vi "Actor Core.vi"(8 "error in":errorcluster, 11 "Meter in":refnum<class "Meter.lvclass">) -> (0 "error out":errorcluster, 3 "Actor out":refnum<class "Actor.lvclass">)   [LabVIEW 2018, in "Meter Actor.lvlib" / "Meter.lvclass"]
doc: "(<B>Filename</B>: Actor Framework.lvlib:Actor.lvclass:Actor Core.vi)\n\nReceives messages to the actor, reacts to them, and initiates any error handling that may shut the actor down.\n\nDescendant classes may override this VI to append parallel tasks for the actor to complete while it handles messages. Overrides use the Call Parent Method node."
uses:
  Meter.lvclass
  C:/Users/Administrator/Desktop/2018LabVIEW EMS/EMS Generic Actor/EMS Generic/EMS Generic.lvclass
  <vilib>/ActorFramework/Actor/Actor.lvclass
  EMS Generic Actor/EMS Generic/EMS Generic.lvclass/EMS Generic.ctl
  <vilib>/ORNL/CSEISMIC DDS/CSEISMIC DDS Base/CSEISMIC DDS.lvclass/CSEISMIC DDS.ctl
  <vilib>/ORNL/CSEISMIC DDS/CSEISMIC DDS Base/Accessors/Write DDS Reference.vi
  <vilib>/ORNL/CSEISMIC DDS/CSEISMIC DDS Base/Accessors/Read DDS Reference.vi
  <vilib>/ORNL/CSEISMIC DDS/DDS Reader/DDS Reader.lvclass
  C:/Program Files (x86)/National Instruments/LabVIEW 2018/vi.lib/ORNL/CSEISMIC DDS/CSEISMIC DDS Base/CSEISMIC DDS.lvclass
  <vilib>/ORNL/CSEISMIC DDS/CSEISMIC DDS Base/Error Handler.vi
  Device DDS Communications Framework/Device DDS Communications/Device DDS Communications.lvclass
  EMS Generic Actor/EMS Generic/EMS Generic.lvclass
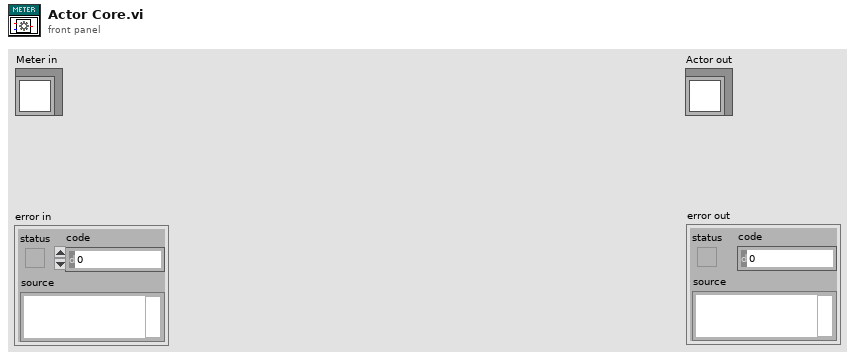
[diagram p1: front panel]
types:
  T1 = typedef "CSEISMIC DDS.lvlib/CSEISMIC DDS.lvclass/DeviceID.ctl" = string
  T2 = typedef "CSEISMIC DDS.lvlib/CSEISMIC DDS.lvclass/Meter_Measurement.ctl" = cluster{"DeviceID":T1, "Voltage":dbl[], "Current":dbl[], "RealPower":dbl[], "ReactivePower":dbl[], "LineConfig":u8[], "Frequency":dbl}
  T3 = typedef "LVDDS_library.lvlib/DDS Sample Info.ctl" = cluster{"DDS_SampleStateKind":enum32{"DDS_INVALID_SAMPLE_STATE", "DDS_READ_SAMPLE_STATE", "DDS_NOT_READ_SAMPLE_STATE"}, "DDS_ViewStateKind":enum32{"DDS_INVALID_SAMPLE_STATE", "DDS_NEW_VIEW_STATE", "DDS_NOT_NEW_VIEW_STATE"}, "DDS_InstanceStateKind":enum32{"DDS_INVALID_STATE", "DDS_ALIVE_INSTANCE_STATE", "DDS_NOT_ALIVE_DISPOSED_INSTANCE_STATE", "", "DDS_NOT_ALIVE_NO_WRITERS_INSTANCE_STATE"}, "sec":i32, "nanosec":u32, "valid_data":bool}
  T4 = typedef "CSEISMIC DDS.lvlib/CSEISMIC DDS.lvclass/Meter_Info.ctl" = cluster{"DeviceID":T1, "LineConfig":u8[], "NominalVoltage(V)":dbl}
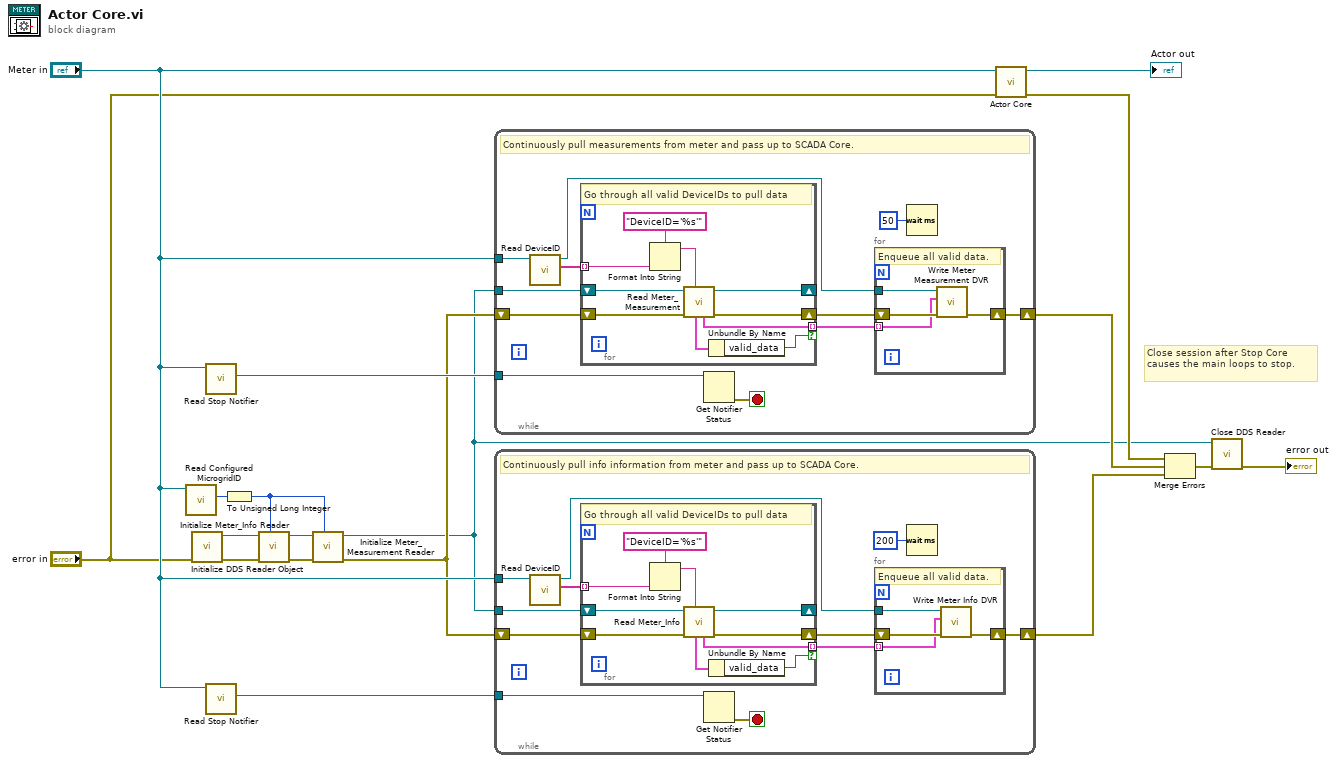
[diagram p0: block diagram]
diagram:
  # "Close session after Stop Core causes the main loops to stop."
  n1 = call "Read Configured MicrogridID.vi"("EMS Generic in"="Meter in") -> ("Microgrid ID"=w18:u8)  [unwired: 8 in, 2 out]
  n2 = call <vilib>:"Initialize DDS Reader Object.vi"("error in"="error in") -> ("error out"=w12:errorcluster, "DDS Reader out"=w11:refnum<class "DDS Reader.lvclass">)  [unwired: 9 in]
  n3 = call "Read Stop Notifier.vi"("EMS Generic in"="Meter in") -> ("stop"=w14:refnum<notifier>)  [unwired: 9 in, 1 out]
  n4 = call "Read Stop Notifier.vi"("EMS Generic in"="Meter in") -> ("stop"=w7:refnum<notifier>)  [unwired: 9 in, 1 out]
  n5 = To Unsigned Long Integer(number=w18) -> (unsigned 32bit integer=w9:u32)
  n6 = call <vilib>:"Initialize Meter_Info Reader.vi"("MicrogridID"=w9, "error in"=w12, "DDS Reader in"=w11) -> ("error out"=w13:errorcluster, "DDS Reader out"=w10:refnum<class "DDS Reader.lvclass">)  [unwired: 7 in]
  n7 = call <vilib>:"Initialize Meter_Measurement Reader.vi"("MicrogridID"=w9, "error in"=w13, "DDS Reader in"=w10) -> ("error out"=w5:errorcluster, "DDS Reader out"=w4:refnum<class "DDS Reader.lvclass">)  [unwired: 7 in]
  n8 = while {
    tunnel: w14 -> [w29]
    shift-right: [w28] -> w17
    shift-left: w5 -> [w23]
    tunnel: "Meter in" -> [w25]
    tunnel: w4 -> [w22]
    stop <- w27 stop-if-true
    # "Continuously pull measurements from meter and pass up to SCADA Core."
    n9 = call-dynamic "Read DeviceID.vi"("Device DDS Communications in"=w25) -> ("DeviceID"=w24:T1[], "Device DDS Communications out"=w19:refnum<class "Meter.lvclass">)  [unwired: 9 in]
    n10 = for {
      shift-right: [w42] -> _
      shift-left: w22 -> [w43]
      shift-right: [w41] -> w21
      shift-left: w23 -> [w40]
      tunnel: w24 -> [w38] mode=indexing
      tunnel: [w35] -> w20 mode=indexing if=w34
      # "Go through all valid DeviceIDs to pull data"
      n11 = Format Into String(format string="DeviceID='%s'", w38) -> (resulting string=w37:string)  [unwired: 2 in, 1 out]
      n12 = call <vilib>:"Read Meter_Measurement.vi"("Query condition"=w37, "error in"=w40, "DDS Reader in"=w43) -> ("error out"=w41:errorcluster, "DDS Reader out"=w42:refnum<class "DDS Reader.lvclass">, "data"=w35:T2, "DDS Sample Info"=w36:T3)  [unwired: 5 in]
      n13 = Unbundle By Name(w36) -> ("valid_data"=w34:bool)
    }
    n14 = Get Notifier Status(notifier=w29) -> (error out=w27:errorcluster)  [unwired: 1 in, 4 out]
    n15 = for {
      shift-right: [w32] -> w28
      shift-left: w21 -> [w33]
      tunnel: w20 -> [w31] mode=indexing
      tunnel: w19 -> [w30]
      # "Enqueue all valid data."
      n16 = call "Write Meter Measurement DVR.vi"("error in"=w33, "Meter_Measurement"=w31, "EMS Generic in"=w30) -> ("error out"=w32:errorcluster)  [unwired: 7 in, 1 out]
    }
    n17 = Wait (ms)(milliseconds to wait=u32 50) -> ()  [unwired: 1 out]
  }
  n18 = while {
    tunnel: w7 -> [w54]
    shift-right: [w53] -> w3
    shift-left: w5 -> [w48]
    tunnel: "Meter in" -> [w50]
    tunnel: w4 -> [w47]
    stop <- w52 stop-if-true
    # "Continuously pull info information from meter and pass up to SCADA Core."
    n19 = call-dynamic "Read DeviceID.vi"("Device DDS Communications in"=w50) -> ("DeviceID"=w49:T1[], "Device DDS Communications out"=w44:refnum<class "Meter.lvclass">)  [unwired: 9 in]
    n20 = for {
      shift-right: [w67] -> _
      shift-left: w47 -> [w68]
      shift-right: [w66] -> w46
      shift-left: w48 -> [w65]
      tunnel: w49 -> [w63] mode=indexing
      tunnel: [w60] -> w45 mode=indexing if=w59
      # "Go through all valid DeviceIDs to pull data"
      n21 = Format Into String(format string="DeviceID='%s'", w63) -> (resulting string=w62:string)  [unwired: 2 in, 1 out]
      n22 = call <vilib>:"Read Meter_Info.vi"("Query condition"=w62, "error in"=w65, "DDS Reader in"=w68) -> ("error out"=w66:errorcluster, "DDS Reader out"=w67:refnum<class "DDS Reader.lvclass">, "data"=w60:T4, "DDS Sample Info"=w61:T3)  [unwired: 5 in]
      n23 = Unbundle By Name(w61) -> ("valid_data"=w59:bool)
    }
    n24 = Get Notifier Status(notifier=w54) -> (error out=w52:errorcluster)  [unwired: 1 in, 4 out]
    n25 = for {
      shift-right: [w57] -> w53
      shift-left: w46 -> [w58]
      tunnel: w45 -> [w56] mode=indexing
      tunnel: w44 -> [w55]
      # "Enqueue all valid data."
      n26 = call "Write Meter Info DVR.vi"("error in"=w58, "Meter_Info"=w56, "EMS Generic in"=w55) -> ("error out"=w57:errorcluster)  [unwired: 7 in, 1 out]
    }
    n27 = Wait (ms)(milliseconds to wait=u32 200) -> ()  [unwired: 1 out]
  }
  n28 = call-parent "Actor Core.vi"("error in"="error in", "Actor in"="Meter in") -> ("error out"=w16:errorcluster, "Actor out"=→"Actor out":refnum<class "Actor.lvclass">)  [unwired: 8 in]
  n29 = Merge Errors(w16, w17, w3) -> (w2:errorcluster)
  n30 = call <vilib>:"Close DDS Reader.vi"("error in"=w2, "DDS Reader in"=w4) -> ("error out"=→"error out":errorcluster)  [unwired: 9 in]
